vi "Test Process Retains State when stopped.vi"(8 "error in (no error)":errorcluster, 11 "Process Test In":refnum<class "Process Test.lvclass">) -> (0 "error out":errorcluster, 3 "Process Test Out":refnum<class "Process Test.lvclass">)   [LabVIEW 2020, in "Process Test.lvclass"]
uses:
  Process Test.lvclass
  <vilib>/Asteme/LUnit/Test Case.lvclass
  Mock Error Handler/Mock Error Handler.lvclass
  Framework/Process/Process.lvclass
  C:/Users/anton/Documents/GitHub/Triarc-Framework/source/Framework Test/Base Class Test/Base Class Test.lvclass
  C:/Program Files (x86)/National Instruments/LabVIEW 2020/vi.lib/Asteme/LUnit/Test Case.lvclass
  C:/Users/anton/Documents/GitHub/Triarc-Framework/source/Framework Test/Process Test/Process Test.lvclass
  C:/Users/anton/Documents/GitHub/Triarc-Framework/source/Framework/Process/Process.lvclass
  C:/Users/anton/Documents/GitHub/Triarc-Framework/source/Framework/Base/Base.lvclass
  C:/Users/anton/Documents/GitHub/Triarc-Framework/source/Framework/Configuration File/Configuration File.lvclass
  C:/Users/anton/Documents/GitHub/Triarc-Framework/source/Framework Test/Mock Error Handler/Mock Error Handler.lvclass
  C:/Users/anton/Documents/GitHub/Triarc-Framework/source/Framework/Error Handler Interface/Error Handler Interface.lvclass
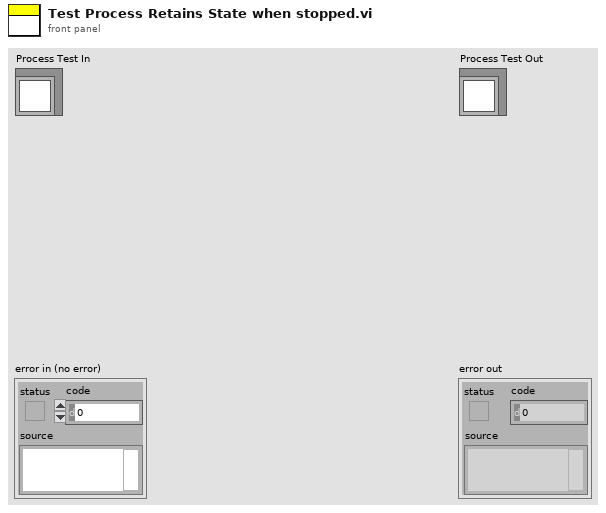
[diagram p1: front panel]
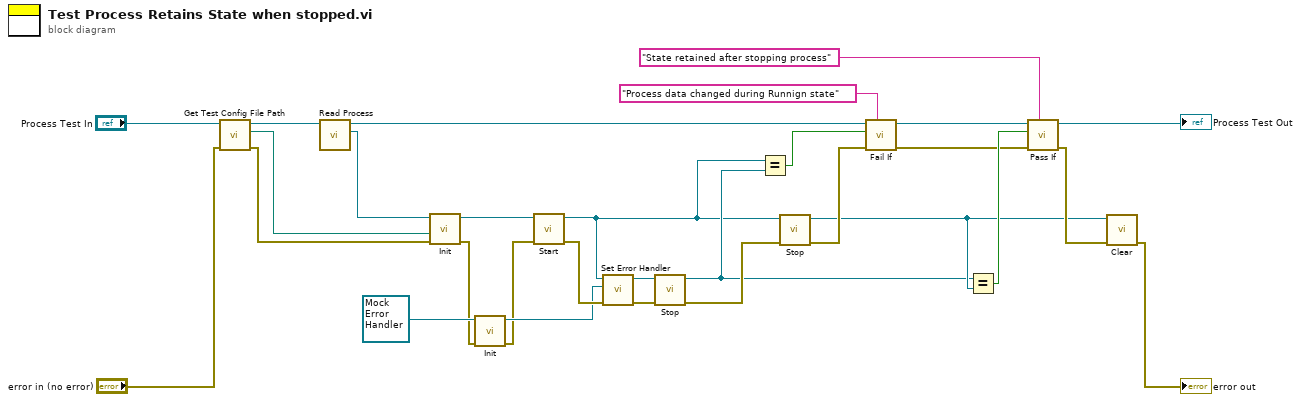
[diagram p0: block diagram]
diagram:
  n1 = call-dynamic "Get Test Config File Path.vi"("error in (no error)"="error in (no error)", "Base Class Test in"="Process Test In") -> ("error out"=w26:errorcluster, "Test config path"=w28:path, "Base Class Test out"=w29:refnum<class "Process Test.lvclass">)  [unwired: 7 in]
  n2 = call "Read Process.vi"("Process Test in"=w29) -> ("Process.lvclass"=w27:refnum<class "Process.lvclass">, "Process Test out"=w6:refnum<class "Process Test.lvclass">)  [unwired: 8 in, 1 out]
  n3 = call-dynamic "Init.vi"("error in (no error)"=w26, "Config File Path"=w28, "Process In"=w27) -> ("error out"=w16:errorcluster, "Process Out"=w20:refnum<class "Process.lvclass">)  [unwired: 7 in]
  n4 = call-dynamic "Init.vi"("error in (no error)"=w16, "Mock Error Handler In"=refnum<class "Mock Error Handler.lvclass"> refnum ("Mock Error Handler.lvclass")) -> ("error out"=w15:errorcluster, "Mock Error Handler Out"=w17:refnum<class "Mock Error Handler.lvclass">)  [unwired: 8 in]
  n5 = call "Start.vi"("error in (no error)"=w15, "Process In"=w20) -> ("error out"=w21:errorcluster, "Process Out"=w3:refnum<class "Process.lvclass">)  [unwired: 8 in]
  n6 = call "Set Error Handler.vi"("error in (no error)"=w21, "Error Handler"=w17, "Process In"=w3) -> ("error out"=w9:errorcluster, "Process Out"=w12:refnum<class "Process.lvclass">)  [unwired: 7 in]
  n7 = call "Stop.vi"("error in (no error)"=w9, "Process In"=w12) -> ("error out"=w8:errorcluster, "Process Out"=w4:refnum<class "Process.lvclass">)  [unwired: 7 in, 1 out]
  n8 = Equal?(x=w3, y=w4) -> (x = y?=w2:bool)
  n9 = call "Stop.vi"("error in (no error)"=w8, "Process In"=w3) -> ("error out"=w11:errorcluster, "Process Out"=w10:refnum<class "Process.lvclass">)  [unwired: 7 in, 1 out]
  n10 = call <vilib>:"Fail If.vi"("Description"="Process data changed during Runnign state", "error in (no error)"=w11, "Fail?"=w2, "Test Case In"=w6) -> ("error out"=w7:errorcluster, "Test Case Out"=w5:refnum<class "Process Test.lvclass">)  [unwired: 6 in]
  n11 = Equal?(x=w4, y=w10) -> (x = y?=w18:bool)
  n12 = call <vilib>:"Pass If.vi"("Description"="State retained after stopping process", "error in (no error)"=w7, "Pass?"=w18, "Test Case In"=w5) -> ("error out"=w14:errorcluster, "Test Case Out"=→"Process Test Out":refnum<class "Process Test.lvclass">)  [unwired: 6 in]
  n13 = call-dynamic "Clear.vi"("error in (no error)"=w14, "Process In"=w10) -> ("error out"=→"error out":errorcluster)  [unwired: 8 in, 1 out]
